vi "Write Default Configuration Path.vi"(5 "Default Configuration Path":path, 9 "PythonConfiguration in":refnum<class "PythonConfiguration.lvclass">) -> (3 "PythonConfiguration out":refnum<class "PythonConfiguration.lvclass">)   [LabVIEW 2014, in "PythonConfiguration.lvclass"]
uses:
  PythonConfiguration.lvclass
  PythonConfiguration.lvclass/PythonConfiguration.ctl
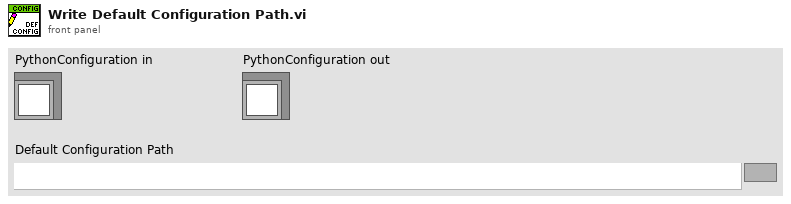
[diagram p1: front panel]
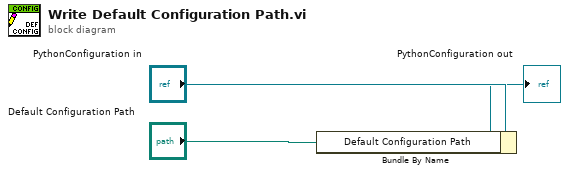
[diagram p0: block diagram]
diagram:
  n1 = Bundle By Name(cluster="PythonConfiguration in", "Default Configuration Path"="Default Configuration Path") -> (→"PythonConfiguration out":refnum<class "PythonConfiguration.lvclass">)
